vi "ADXL345_Init.vi"(2 "error in":errorcluster, 3 "Range (± 4g)":enum16{"± 2g", "± 4g", "± 8g", "± 16g"}(ring)=enum."± 8g", 4 "Arduino Resource":T1={"VISA resource"="", "Board Type"=enum."Uno", "Connection Type"=enum."USB / Serial", "Bytes Per Packet (15)"=15}) -> (0 "error out":errorcluster, 1 "Arduino Resource":T1={"VISA resource"="", "Board Type"=enum."Uno", "Connection Type"=enum."USB / Serial", "Bytes Per Packet (15)"=15})   [LabVIEW 2012]
uses:
  <vilib>/LabVIEW Interface for Arduino/Type Defs/Arduino Resource.ctl
  <vilib>/LabVIEW Interface for Arduino/Type Defs/Board Type.ctl
  <vilib>/LabVIEW Interface for Arduino/LabVIEW Interface for Arduino.lvlib
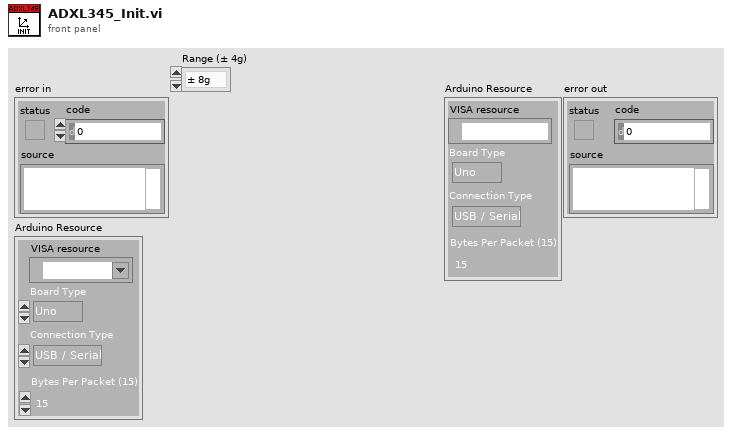
[diagram p1: front panel]
types:
  T1 = typedef "LabVIEW Interface for Arduino.lvlib/Arduino Resource.ctl" = cluster{"VISA resource":refnum<visa-resource-name>, "Board Type":T2, "Connection Type":enum8{"USB / Serial"}, "Bytes Per Packet (15)":u8}
  T2 = typedef "LabVIEW Interface for Arduino.lvlib/Board Type.ctl" = enum16{"Uno", "Dimuelanove w/Atmega 328", "Mega 2560"}
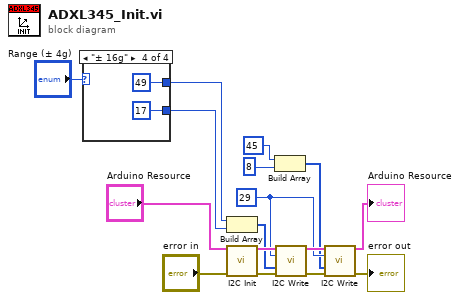
[diagram p0: block diagram]
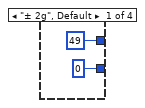
[diagram p2: hidden frame]
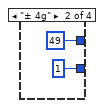
[diagram p3: hidden frame]
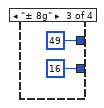
[diagram p4: hidden frame]
diagram:
  w8 = u8 29 ("Address (0)")
  n1 = case shown="\"± 16g\"" "Range (± 4g)" {
    tunnel: [u8 49 ("element") u8 49 ("element") u8 49 ("element") u8 49 ("element")] -> w2
    tunnel: [u8 0 ("element") u8 1 ("element") u8 16 ("element") u8 17 ("element")] -> w1
    frame "± 2g", Default {
    }
    frame "± 4g" {
    }
    frame "± 8g" {
    }
    frame "± 16g" {
    }
  }
  n2 = Build Array(w2, w1) -> (w4:u8[])
  n3 = call <vilib>:"I2C Init.vi"("Arduino Resource"="Arduino Resource", "error in"="error in") -> ("Arduino Resource"=w16:T1, "error out"=w11:errorcluster)  [unwired: 12 in]
  n4 = Build Array(u8 45 ("element"), u8 8 ("element")) -> (w7:u8[])
  n5 = call <vilib>:"I2C Write.vi"("Arduino Resource"=w16, "Address (0)"=w8, "I2C Data Bytes"=w4, "error in"=w11) -> ("Arduino Resource"=w15:T1, "error out"=w12:errorcluster)  [unwired: 10 in]
  n6 = call <vilib>:"I2C Write.vi"("Arduino Resource"=w15, "Address (0)"=w8, "I2C Data Bytes"=w7, "error in"=w12) -> ("Arduino Resource"=→"Arduino Resource":T1, "error out"=→"error out":errorcluster)  [unwired: 10 in]
